vi "Excel class path.vi"() -> (8 "Excel class path":path)   [LabVIEW 2017, in "NI_ReportGenerationCore.lvlib"]
uses:
  <vilib>/Utility/NIReport.llb/NI_ReportGenerationCore.lvlib
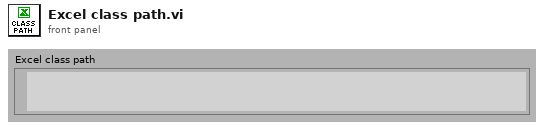
[diagram p1: front panel]
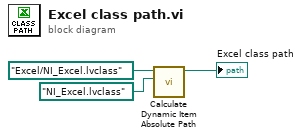
[diagram p0: block diagram]
diagram:
  n1 = call <vilib>:"Calculate Dynamic Item Absolute Path.vi"("Compat Built App Relative Path"=path "NI_Excel.lvclass" ("path"), "Core Relative Path"=path "Excel/NI_Excel.lvclass" ("path")) -> ("Resulting Absolute Path"=→"Excel class path":path)  [unwired: 9 out]
